vi "Parse Response JSON.vi"(8 "error in (no error)":errorcluster, 10 "Response JSON":string, 11 "RGetSceneItemID in":refnum<class "RGetSceneItemID.lvclass">) -> (0 "error out":errorcluster, 3 "RGetSceneItemID out":refnum<class "RGetSceneItemID.lvclass">)   [LabVIEW 2020, in "obs-websocket.lvlib" / "RGetSceneItemID.lvclass"]
uses:
  RGetSceneItemID.lvclass
  RGetSceneItemID.lvclass/RGetSceneItemID.ctl
  69081c51-f27d-418b-89ce-df9272e6827d.vi
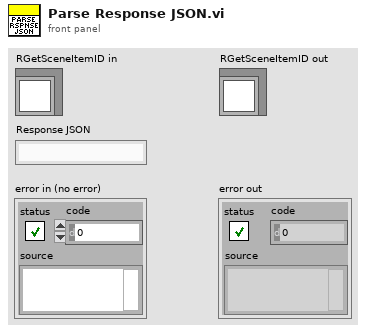
[diagram p1: front panel]
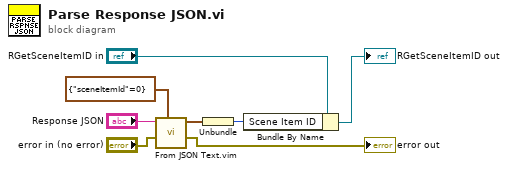
[diagram p0: block diagram]
diagram:
  n1 = call "From JSON Text.vim"("Data Type and Default Value"=cluster{"sceneItemId":i32} {"sceneItemId"=0}, "error in (no error)"="error in (no error)", "JSON"="Response JSON") -> ("error out"=→"error out":errorcluster, "Data out"=w2:cluster{"sceneItemId":i32})  [unwired: 7 in]
  n2 = Unbundle(w2) -> ("sceneItemId"=w1:i32)
  n3 = Bundle By Name(cluster="RGetSceneItemID in", "Scene Item ID"=w1) -> (→"RGetSceneItemID out":refnum<class "RGetSceneItemID.lvclass">)
